vi "Count Up.vi"(11 "Reset":bool) -> (3 "Out (I32)":i32)   [LabVIEW 2014]
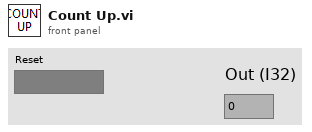
[diagram p1: front panel]
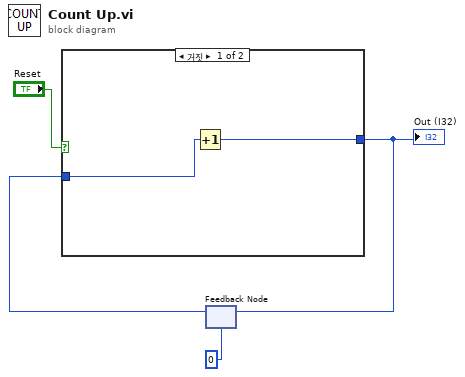
[diagram p0: block diagram]
diagram:
  n1 = feedback #1(0) -> (w2:i32)
  n2 = case shown="거짓" "Reset" {
    tunnel: [w6 _] -> w3
    tunnel: w2 -> [w5 _]
    frame False {
      n3 = Increment(x=w5) -> (x+1=w6:i32)
    }
    frame True {
    }
  }
  "Out (I32)" <- w3
  n4 = feedback-in #1(w3) -> ()
